vi "UpdateSelectColor.vi"(7 "Available Points":refnum<vi>, 8 "error in (no error)":errorcluster, 10 "Available Points Idx":T1) -> (0 "error out":errorcluster)   [LabVIEW 2019]
uses:
  <vilib>/Utility/miscctls.llb/LVRowAndColumnTypeDef.ctl
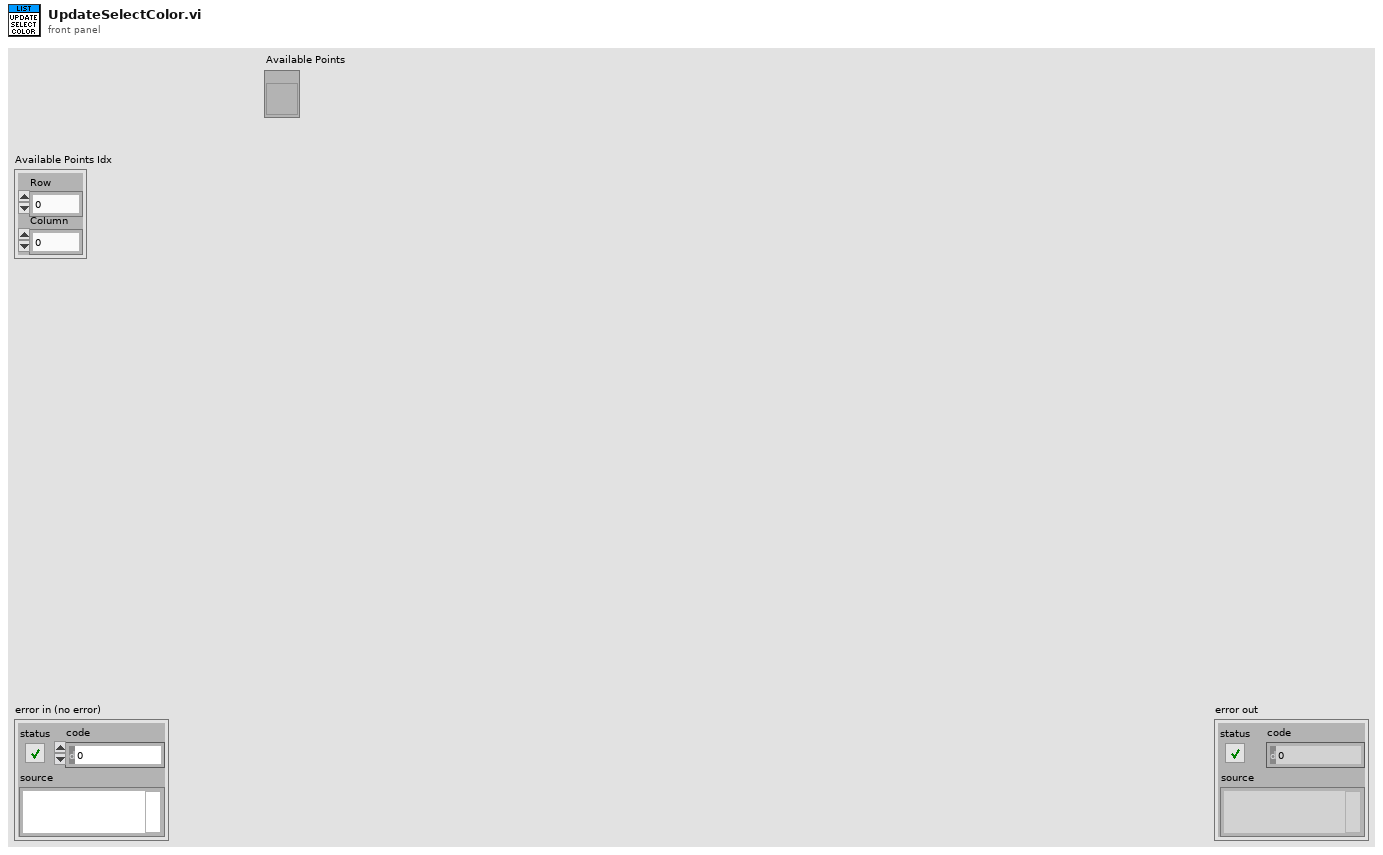
[diagram p1: front panel]
types:
  T1 = typedef "LVRowAndColumnTypeDef.ctl" = cluster{"Row":i32, "Column":i32}
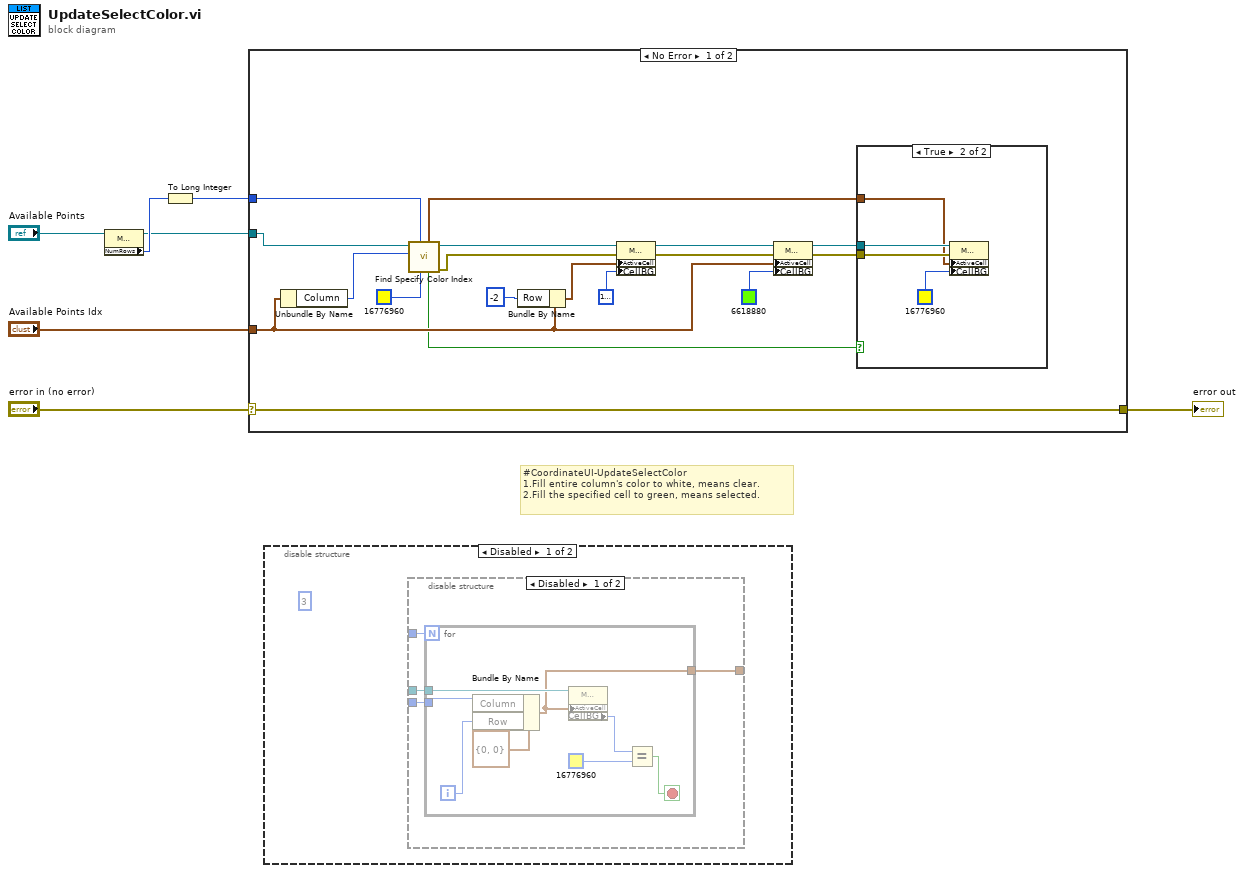
[diagram p0: block diagram]
diagram:
  # "#CoordinateUI-UpdateSelectColor\n1.Fill entire column's color to white, means clear.\n2.Fill the specified cell to green, means selected."
  n1 = property class="MCListbox (strict)"(reference="Available Points") -> (reference out=w2:refnum<vi>, "NumRows"=w5:u32)  [unwired: 1 in, 1 out]
  n2 = To Long Integer(number=w5) -> (32bit integer=w1:i32)
  n3 = case shown="No Error" "error in (no error)" {
    selector: "error in (no error)" -> [w20 w30]
    tunnel: "Available Points Idx" -> [w12 _]
    tunnel: [w20 w30] -> w6
    tunnel: w2 -> [w15 _]
    tunnel: w1 -> [w14 _]
    frame No Error {
      n4 = Unbundle By Name(w12) -> ("Column"=w11:i32)
      n5 = call "Find Specify Color Index.vi"("Color Box"=u32 16776960, "Num of Row"=w14, "Column"=w11, "MultiList Ref In"=w15) -> ("error out"=w13:errorcluster, "MultiList Ref Out"=w16:refnum<vi>, "Exist?"=w9:bool, "Active Cell"=w8:T1)  [unwired: 3 in, 1 out]
      n6 = Bundle By Name(cluster=w12, "Row"=-2) -> (w23:T1)
      n7 = property class="MCListbox (strict)"(reference=w16, error in=w13, "ActiveCell"=w23, "CellBG"=u32 16777225) -> (reference out=w25:refnum<vi>, error out=w18:errorcluster)
      n8 = property class="MCListbox (strict)"(reference=w25, error in=w18, "ActiveCell"=w12, "CellBG"=u32 6618880) -> (reference out=w19:refnum<vi>, error out=w17:errorcluster)
      n9 = case shown="True" w9 {
        tunnel: w19 -> [_ w29]
        tunnel: w17 -> [_ w28]
        tunnel: w8 -> [_ w26]
        frame False {
        }
        frame True {
          n10 = property class="MCListbox (strict)"(reference=w29, error in=w28, "ActiveCell"=w26, "CellBG"=u32 16776960) -> ()  [unwired: 2 out]
        }
      }
    }
    frame Error {
    }
  }
  "error out" <- w6
  n11 = disable-structure shown="Disabled" {
    frame Disabled {
      (unwired) 3
      n12 = disable-structure shown="Disabled" {
        disable-tunnel: _ -> [w34 _]
        disable-tunnel: _ -> [w33 _]
        disable-tunnel: _ -> [w32 _]
        disable-tunnel: [w31 _] -> _
        frame Disabled {
          n13 = for {
            N: w33 -> [_]
            tunnel: w34 -> [w37]
            tunnel: w32 -> [w36]
            tunnel: [w35] -> w31
            i -> [w39]
            stop <- w38 stop-if-true
            n14 = Bundle By Name(cluster=T1 {"Row"=0, "Column"=0} ("Active Cell:Active Cell"), "Column"=w36, "Row"=w39) -> (w35:T1)
            n15 = property class="MCListbox (strict)"(reference=w37, "ActiveCell"=w35) -> ("CellBG"=w41:u32)  [unwired: 1 in, 2 out]
            n16 = Equal?(x=w41, y=u32 16776960) -> (x = y?=w38:bool)
          }
        }
        frame Enabled {
        }
      }
    }
    frame Enabled {
    }
  }
